vi "SAW_Jeremy.vi"() -> ()   [LabVIEW 2020]
panel:
  out "S11":dbl[][](graph)
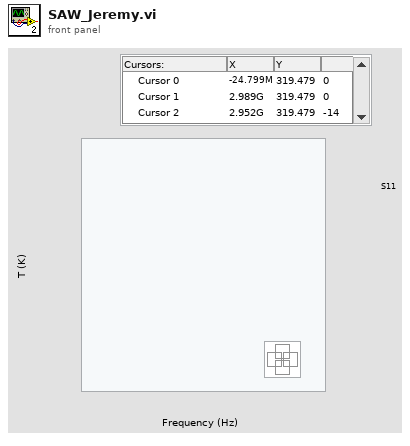
[diagram p1: front panel]
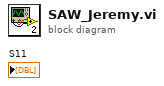
[diagram p0: block diagram]
diagram:
